vi "20170411-lecture3-global variable.vi"() -> ()   [LabVIEW 2014]
panel:
  out "run status":bool
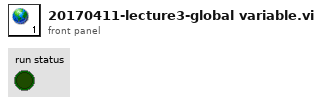
[diagram p1: front panel]
diagram:
